vi "ALTS-2015 wait.vi"(8 "error in":errorcluster, 10 "Wait (s)":dbl format="%.4f", 11 "Start time":timestamp) -> (0 "error out":errorcluster, 2 "Passed time (s)":dbl, 3 "Timed out? / Estop?":bool)   [LabVIEW 2013]
panel:
  # "Inputs"
  # "Outputs"
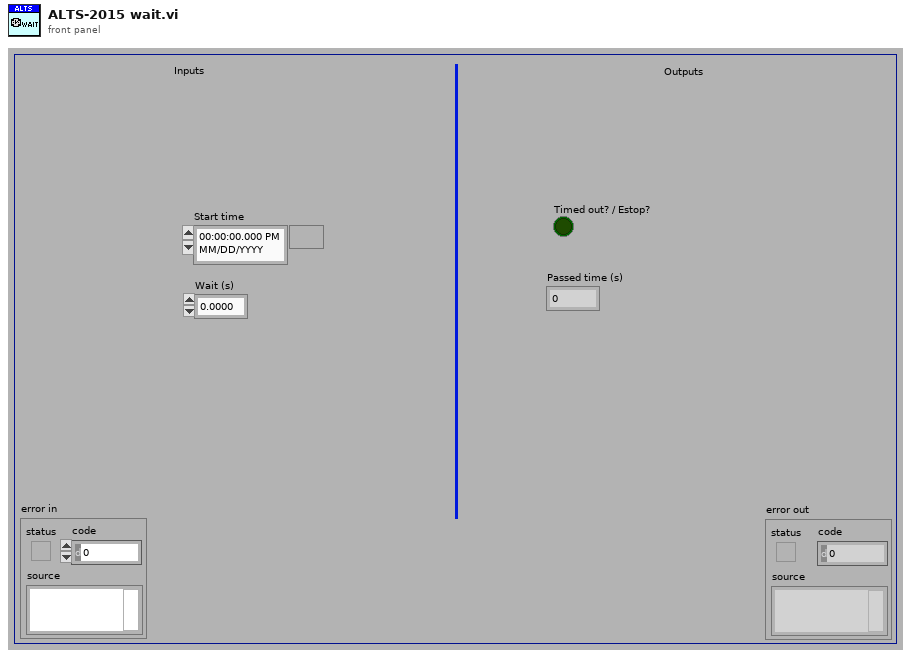
[diagram p1: front panel]
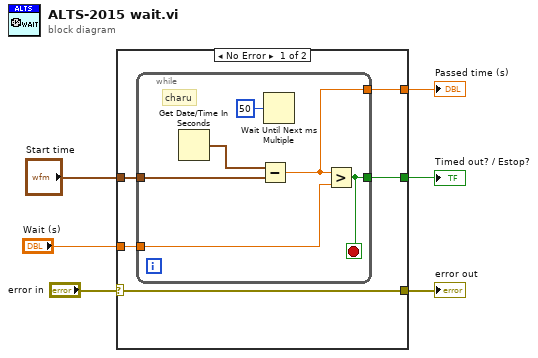
[diagram p0: block diagram]
diagram:
  n1 = case shown="No Error" "error in" {
    selector: "error in" -> [w11 w20]
    tunnel: [w11 w20] -> w5
    tunnel: "Start time" -> [w10 _]
    tunnel: "Wait (s)" -> [w9 _]
    tunnel: [w8 TRUE] -> w3
    tunnel: [w7 u32 0] -> w2
    frame No Error {
      n2 = while {
        tunnel: w10 -> [w17]
        tunnel: w9 -> [w16]
        tunnel: [w13] -> w8
        tunnel: [w14] -> w7
        stop <- w13 stop-if-true
        # "charu"
        n3 = Get Date/Time In Seconds() -> (seconds since 1Jan1904=w15:timestamp)
        n4 = Subtract(x=w15, y=w17) -> (x-y=w14:dbl)
        n5 = Wait Until Next ms Multiple(millisecond multiple=u32 50) -> ()  [unwired: 1 out]
        n6 = Greater?(x=w14, y=w16) -> (0:w13:bool)
      }
    }
    frame Error {
    }
  }
  "error out" <- w5
  "Timed out? / Estop?" <- w3
  "Passed time (s)" <- w2
